vi "stimulus_builder.vi"() -> ()   [LabVIEW 2012]
uses:
  Trace controls.ctl
  probe_point.ctl
  arb_stimulus_kind.ctl
  <vilib>/Platform/TimedLoop/XDataNode/timing_clust.ctl
  <vilib>/Platform/TimedLoop/XDataNode/nitl_modes.ctl
  <vilib>/Platform/TimedLoop/XDataNode/wakeup.ctl
  <vilib>/Analysis/Matrix/Numeric/Conversions/Array To Matrix.vi
  <vilib>/Analysis/Matrix/Numeric/Conversions/Array To Matrix - RA.vi
  <vilib>/Platform/TimedLoop/XDataNode/XDataNode.xnode
  <vilib>/Platform/TimedLoop/XDataNode/XDNodeRunTimeDep.lvlib
panel:
  in  "Stimulus Z rotation":dbl(slide)=-5.10702591327572e-15 min=-90.0 max=90.0 scale=-90.0..90.0
  in  "Normalize":bool
  in  "Bandwidth":dbl=inf format="%0.3f"
  in  "Detrend":bool
  in  "Negate":bool
  in  "Update":bool
  in  "Append reversed":bool
  out "New stimulus":sgl[][](array[numeric]) format="%#_4g"
  out "2D position":cluster{sgl[], sgl[]}[](graph)
  in  "Parameters":sgl[](array[numeric]) format="%#_4p"
  in  "Kind":T1
  in  "Signal file path":path
  in  "Trace controls":T2[](array[typedef])=[{"+ stim"=FALSE, "Relative"=TRUE, "Scale"=enum."1X", "Probe point"=enum."Handle origin", "XYZ selector"={"Boolean"=TRUE, "Boolean 2"=TRUE, "Boolean 3"=TRUE}, "To tip"=FALSE}, {"+ stim"=FALSE, "Relative"=TRUE, "Scale"=enum."1X", "Probe point"=enum."Handle angles", "XYZ selector"={"Boolean"=TRUE, "Boolean 2"=TRUE, "Boolean 3"=TRUE}, "To tip"=FALSE}, {"+ stim"=FALSE, "Relative"=FALSE, "Scale"=enum."1X", "Probe point"=enum."Position (tip)", "XYZ selector"={"Boolean"=FALSE, "Boolean 2"=FALSE, "Boolean 3"=FALSE}, "To tip"=FALSE}, {"+ stim"=FALSE, "Relative"=FALSE, "Scale"=enum."1X", "Probe point"=enum."Position (tip)", "XYZ selector"={"Boolean"=FALSE, "Boolean 2"=FALSE, "Boolean 3"=FALSE}, "To tip"=FALSE}]
  in  "Store":bool
  in  "Stop":bool
  in  "Window":T4(ring)
  out "Power Spectral Density (X)":cluster{"f0":dbl, "df":dbl, "magnitude":dbl[]}[](graph) caption="FFT - (RMS)"
  out "Stimulus":waveform(sgl)[](graph)
  # "Alternative step function with zero DC offset that starts and ends at zero.  May be more suitable to spectral analyis."
  # "Length (sec)"
  # "Stimulus is read from a file (on the real-time target.)  Each line in the file is a single stimulus sample, with up to six floating point numbers (space delimited.)"
  # "Swept-sine signal (chirp) where frequency is an exponential function of time"
  # "Length (sec)"
  # "Low corner (Hz)"
  # "High corner (Hz)"
  # "Band-limited Gaussian noise."
  # "Length (sec)"
  # "Low corner (Hz)"
  # "High corner (Hz)"
  # "Spiral with linear spacing (Archimedes) and constant linear velocity."
  # "Radius (mm)"
  # "Spacing (mm)"
  # "Linear vel (mm/sec)"
  # "Store trace data into stimulus.  Handle KF state may be replayed as \"Total pose\" stimulus."
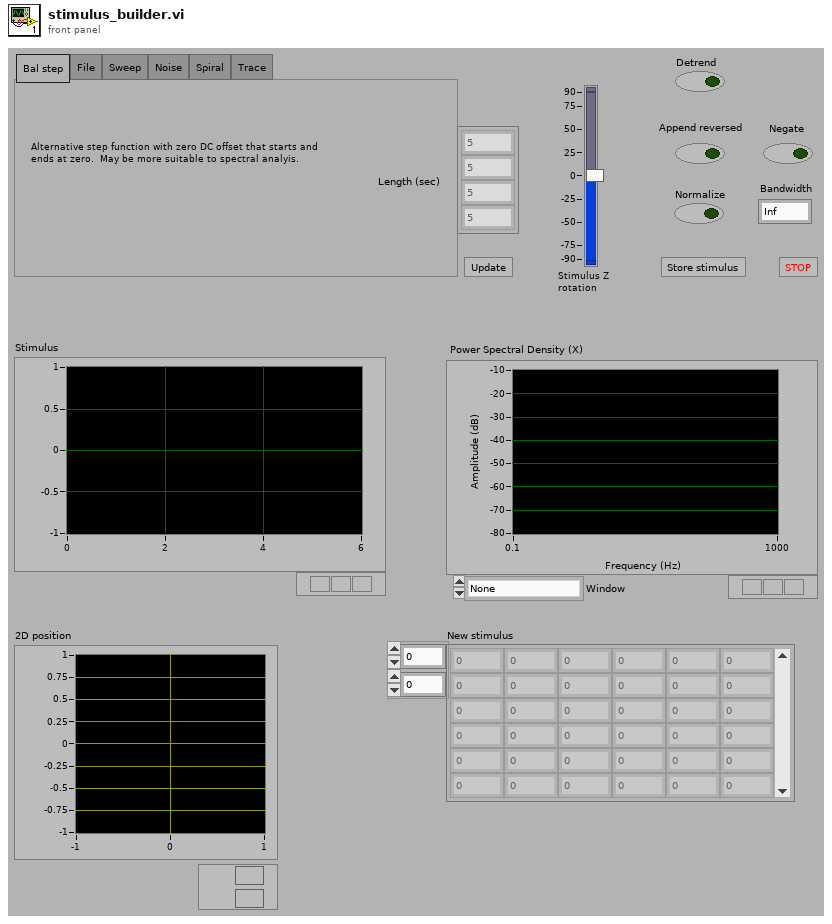
[diagram p1: front panel]
types:
  T1 = typedef "arb_stimulus_kind.ctl" = enum32{"Bal step", "File", "Sweep", "Noise", "Spiral", "Trace"}
  T2 = typedef "Trace controls.ctl" = cluster{"+ stim":bool, "Relative":bool, "Scale":enum16{"1X", "10X", "100X", "1KX", "10KX"}, "Probe point":T3, "XYZ selector":cluster{"Boolean":bool, "Boolean 2":bool, "Boolean 3":bool}, "To tip":bool}
  T3 = typedef "probe_point.ctl" = enum16{"Position (tip)", "Position (RCM)", "Null pos (tip)", "Null pos (RCM)", "V limiter (tip)", "V Limiter (RCM)", "Goal (tip)", "Goal (RCM)", "Link pos 0", "Link pos 1", "KF link pos 0", "KF link pos 1", "Link rate 0", "Link rate 1", "Link residue 0", "Link residue 1", "Link goal 0", "Link goal 1", "Rate limit 0", "Rate limit 1", "Link error 0", "Link error 1", "Controller 0", "Controller 1", "Output 0", "Output 1", "Drive 0", "Drive 1", "Stimulus 0", "Stimulus 1", "Trace data 0", "Trace data 1", "Analog data 0", "Analog data 1", "Status flags", "Light 0", "Light 1", "Light 2", "Light 3", "Light 4", "Light 5", "Goal origin", "Goal rotation 0", "Goal rotation 1", "Goal rotation 2", "Output origin", "Output rotation 0", "Output rotation 1", "Output rotation 2", "Handle origin", "Handle rotation 0", "Handle rotation 1", "Handle rotation 2", "Handle position", "Handle velocity", "Handle acceleration", "Handle angles", "Handle angle rates", "Handle pos residue", "Handle angle residue", "Trace length"}
  T4 = enum16{"None ", "Hanning", "Hamming", "Blackman-Harris", "Exact Blackman", "Blackman", "Flat Top", "4 Term B-Harris ", "7 Term B-Harris", "Low Sidelobe"}
  T5 = typedef "XDNodeRunTimeDep.lvlib/timing_clust.ctl" = cluster{"Expected End [f-1]":u64, "Actual End [f-1]":u64, "Finished Late? [f-1]":bool, "Expected End [i-1]":u64, "Actual End [i-1]":u64, "Finished Late? [i-1]":bool, "Expected Start [i]":u64, "Actual Start [i]":u64, "Expected Start [f]":u64, "Actual Start [f]":u64, "Source Name":string, "Structure Name":string, "Period":i64, "Deadline":i64, "Offset":i64, "Start":i64, "Priority":i32, "Timeout":i32, "Mode":T6, "Wakeup Reason":T7, "Error":errorcluster, "Source Type":string, "Secondary Source Type":string, "Global End Time":u64, "Global Start Time":u64, "Frame Duration":u64, "Iteration Duration":u64, "Assigned CPU":i32, "I/O Scan Engine Mode":u32}
  T6 = typedef "XDNodeRunTimeDep.lvlib/nitl_modes.ctl" = enum32{"No Change", "Process missed periods, maintain original phase", "Discard missed periods, maintain original phase", "Process missed periods, ignore original phase", "Discard missed periods, ignore original phase"}
  T7 = typedef "XDNodeRunTimeDep.lvlib/wakeup.ctl" = enum32{"Normal", "Aborted", "Asynchronous wakeup", "Timing source error", "Timed loop error", "Timeout"}
  T8 = typedef "NI_Matrix.lvlib/RealMatrix.ctl" = dbl[][]
  T9 = cluster{"Kind":T1, "Parameters":sgl[], "Signal file path":path, "Window":enum16{"None ", "Hanning", "Hamming", "Blackman-Harris", "Exact Blackman", "Blackman", "Flat Top", "4 Term B-Harris ", "7 Term B-Harris", "Low Sidelobe"}, "Trace controls":T2[]}
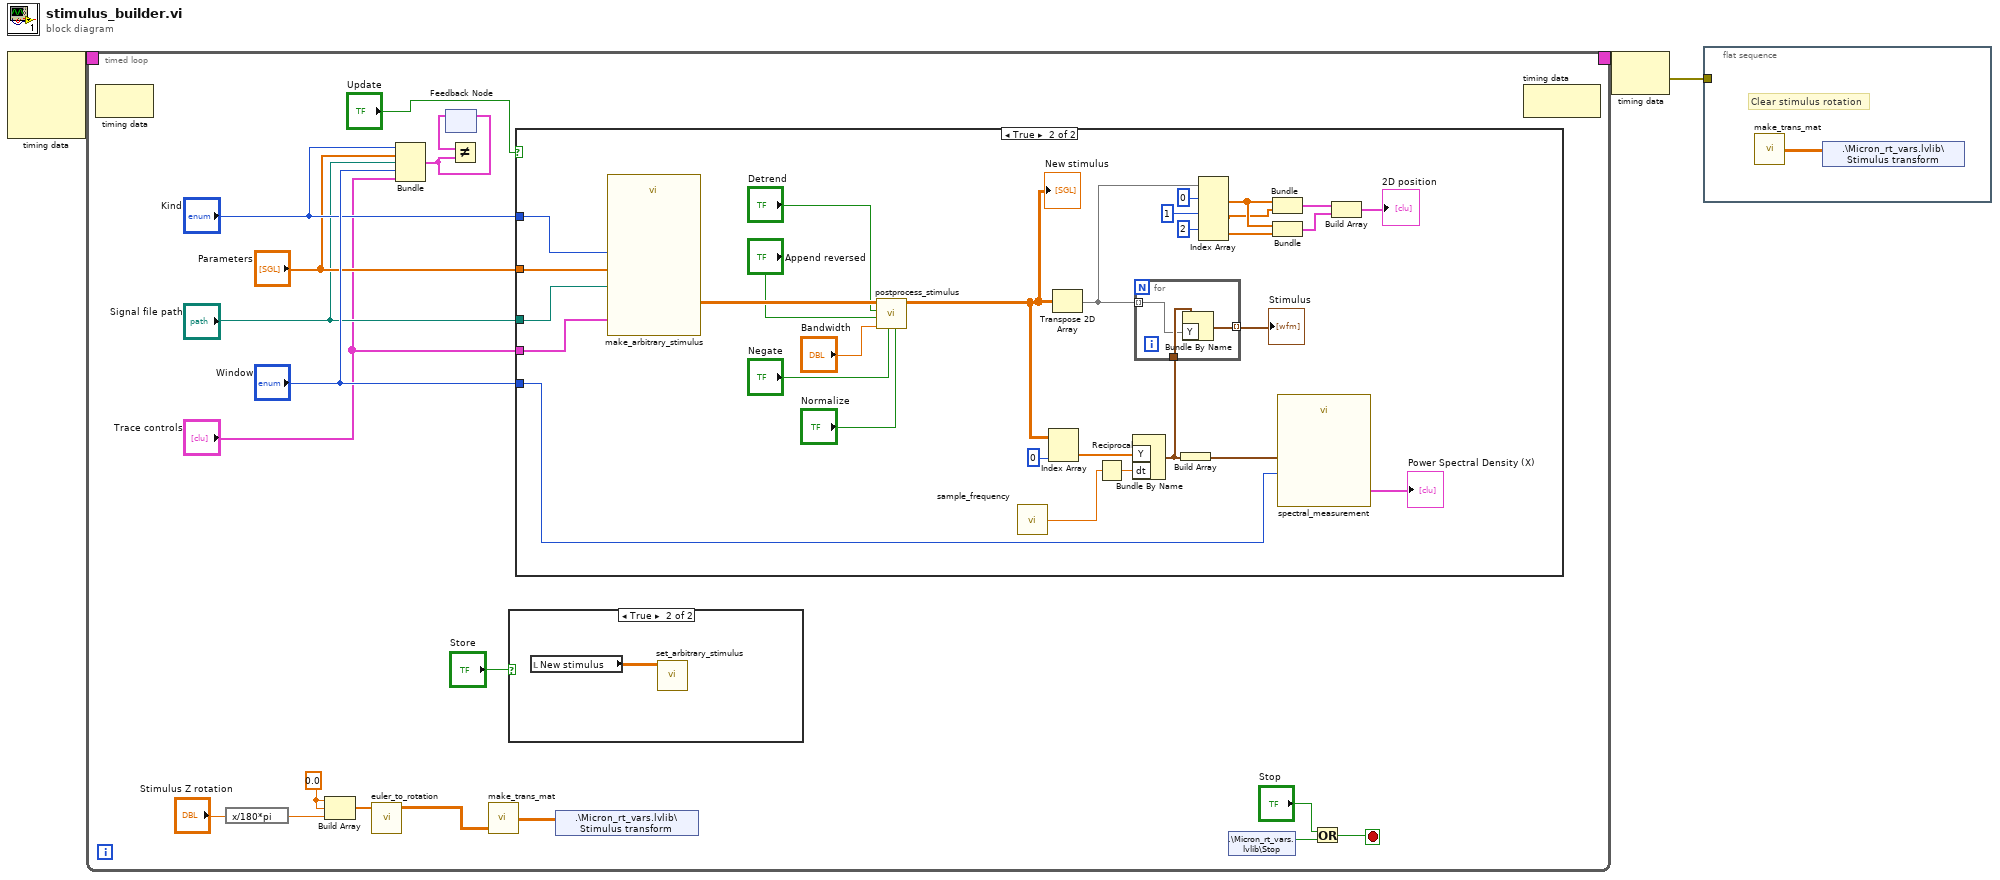
[diagram p0: block diagram]
diagram:
  n1 = node-c288() -> (w3:T5)  [unwired: 4 in]
  n2 = timed-loop {
    timing: w3 -> [_]
    timing-out: [_] -> w2
    stop <- w19 stop-if-true
    w9 = 0.0 ("element")
    n3 = node-c288() -> ()  [unwired: 1 in, 1 out]
    n4 = expression code="x/180*pi"("Stimulus Z rotation") -> (w4:dbl)
    n5 = Build Array(w9, w9, w4) -> (w8:dbl[])
    n6 = call "euler_to_rotation.vi"("Theta XYZ"=w8) -> ("Rotation"=w7:T8)  [unwired: 10 in]
    n7 = Bundle("Kind"="Kind", "Parameters"="Parameters", "Signal file path"="Signal file path", "Window"="Window", "Trace controls"="Trace controls") -> (w16:T9)  [unwired: 1 in]
    n8 = feedback #1() -> (w18:T9)  [unwired: 1 in]
    n9 = feedback-in #1(w16) -> ()
    n10 = Not Equal?(x=w18, y=w16) -> ()  [unwired: 1 out]
    n11 = call "make_trans_mat.vi"("Rotation"=w7) -> ("Transform"=w6:T8)  [unwired: 4 in]
    n12 = case shown="True" "Store" {
      frame False {
      }
      frame True {
        n13 = local read "New stimulus"() -> (w22:sgl[][])
        n14 = call "set_arbitrary_stimulus.vi"("New stimulus"=w22) -> ()  [unwired: 11 in]
      }
    }
    n15 = case shown="True" "Update" {
      tunnel: "Kind" -> [_ w46]
      tunnel: "Parameters" -> [_ w45]
      tunnel: "Signal file path" -> [_ w44]
      tunnel: "Window" -> [_ w43]
      tunnel: "Trace controls" -> [_ w30]
      frame False {
      }
      frame True {
        n16 = call "make_arbitrary_stimulus.vi"("Trace controls"=w30, "Signal file path"=w44, "Parameters"=w45, "Kind"=w46) -> ("Stimulus"=w29:sgl[][])  [unwired: 7 in]
        n17 = call "postprocess_stimulus.vi"("Normalize"="Normalize", "Negate"="Negate", "Bandwidth"="Bandwidth", "Append reversed"="Append reversed", "Detrend"="Detrend", "Input"=w29) -> ("Output"=w28:sgl[][])  [unwired: 5 in]
        "New stimulus" <- w28
        n18 = call "sample_frequency.vi"() -> ("Sample frequency"=w47:dbl)
        n19 = Index Array(array=w28, index (col)=0 ("disabled index (col)")) -> (element=w51:sgl[])  [unwired: 1 in]
        n20 = Transpose 2D Array(2D array=w28) -> (transposed array=w33:sgl[][])
        n21 = Reciprocal(x=w47) -> (1/x=w50:dbl)
        n22 = Bundle By Name("Y"=w51, "dt"=w50) -> (w32:waveform(sgl))  [unwired: 1 out]
        n23 = for {
          tunnel: w33 -> [w54] mode=indexing
          tunnel: w32 -> [w55]
          tunnel: [w53] -> w31 mode=indexing
          n24 = Bundle By Name(cluster=w55, "Y"=w54) -> (w53:waveform(sgl))
        }
        "Stimulus" <- w31
        n25 = Build Array(w32) -> (w49:waveform(sgl)[])
        n26 = Index Array(array=w33, index (row) #1=0 ("index"), index (row) #2=1 ("index"), index (row) #3=2 ("index")) -> (element #1=w36:sgl[], element #2=w35:sgl[], element #3=w34:sgl[])  [unwired: 3 in]
        n27 = Bundle(w36, w35) -> (w41:cluster{sgl[], sgl[]})  [unwired: 1 out]
        n28 = Bundle(w36, w34) -> (w42:cluster{sgl[], sgl[]})  [unwired: 1 out]
        n29 = call "spectral_measurement.vi"("Signals"=w49, "Window"=w43) -> ("PSD"=→"Power Spectral Density (X)":cluster{"f0":dbl, "df":dbl, "magnitude":dbl[]}[])  [unwired: 11 in, 2 out]
        n30 = Build Array(w41, w42) -> (→"2D position":cluster{sgl[], sgl[]}[])
      }
    }
    n31 = shared-variable ".\\Micron_rt_vars.lvlib\\Stimulus transform"(w6) -> ()  [unwired: 2 out]
    n32 = shared-variable ".\\Micron_rt_vars.lvlib\\Stop"() -> (w21:bool)  [unwired: 2 out]
    n33 = Or(x="Stop", y=w21) -> (x .or. y?=w19:bool)
    n34 = node-c288() -> ()  [unwired: 1 in, 1 out]
  }
  n35 = node-c288(w2) -> (w1:errorcluster)
  n36 = flat-sequence {
    tunnel: w1 -> [_]
    frame #0 {
      # "Clear stimulus rotation"
      n37 = call "make_trans_mat.vi"() -> ("Transform"=w58:T8)  [unwired: 5 in]
      n38 = shared-variable ".\\Micron_rt_vars.lvlib\\Stimulus transform"(w58) -> ()  [unwired: 2 out]
    }
  }
